vi "Komponente aus Gasflasche ermitteln.vi"(0 "Referenz Gasflasche":refnum<vi>, 1 "Konzentration IST":dbl, 2 "Wertänderung Gasflasche":bool, 5 "Referenz Komponente":refnum<vi>, 9 "Referenz Konfig Gasflasche":refnum<vi>, 11 "error in (no error)":errorcluster caption="Fehler (Eingang, kein Fehler)") -> (4 "Komponente":string, 6 "Bottle Index":T1 caption="Wert" items=["----"=10000, "IAG NH3 3000"=0, "IAG NH3 200"=1, "IAG NH3 2000"=2, "IAG MG"=3, "IAG O2"=4], 10 "Ausgangs-Cluster":T2, 15 "error out":errorcluster caption="Fehler (Ausgang)")   [LabVIEW 2020, in "System Einstellungen V2.lvlib"]
uses:
  System Einstellungen V2.lvlib
  Gasflasche Auswahl.ctl
  Aktion FGV Gasbottledefinition.ctl
  FT-IR/FGV FT-IR Gasliste Aktionen.ctl
  FT-IR/FT-IR.lvlib
  Gaszuordnung AO/Gaszuordnung AO.lvlib
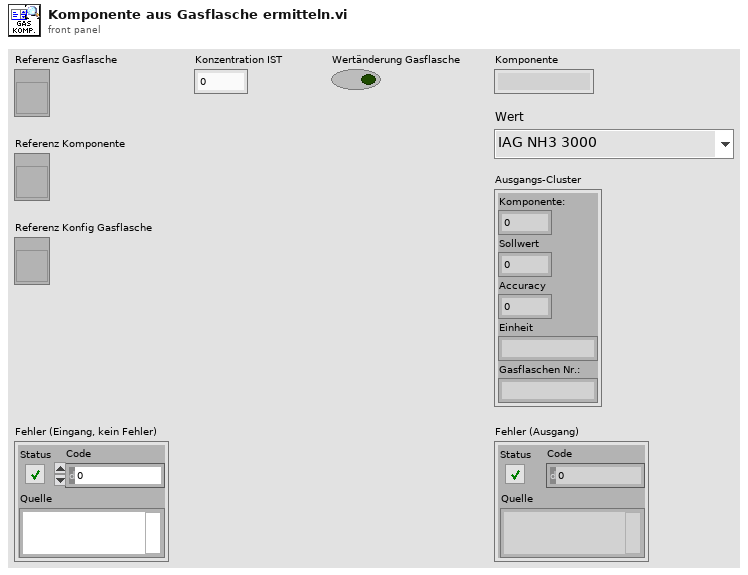
[diagram p1: front panel]
types:
  T1 = typedef "System Einstellungen V2.lvlib/Gasflasche Auswahl.ctl" = u16
  T2 = cluster{"Komponente:":u16, "Sollwert":dbl, "Accuracy":dbl, "Einheit":string, "Gasflaschen Nr.:":string}
  T3 = typedef "FT-IR.lvlib/FGV FT-IR Gasliste Aktionen.ctl" = enum16{"lesen", "Gasliste FT-IR", "Gasliste ausgelesen", "laden", "speichern", "löschen"}
  T4 = typedef "System Einstellungen V2.lvlib/Aktion FGV Gasbottledefinition.ctl" = enum16{"lesen", "schreiben", "löschen", "laden", "speichern", "exportieren", "importieren"}
  T5 = typedef "System Einstellungen V2.lvlib/Gasflasche gesamt.ctl" = cluster{"Gasflasche":T6, "Trägergas":T7, "Komponenten":T8[]}
  T6 = typedef "System Einstellungen V2.lvlib/Gasflasche.ctl" = cluster{"Gasname für die Auswahl":string, "Chargennummer":string, "Ablaufdatum":timestamp}
  T7 = typedef "System Einstellungen V2.lvlib/Traegergas.ctl" = string
  T8 = typedef "System Einstellungen V2.lvlib/Gasflaschenkomponente.ctl" = cluster{"Gasauswahl":string, "Konzentration IST":dbl, "Einheit":string, "Genauigkeit":dbl}
  T9 = typedef "String - Ausgabefeld.ctl" = string
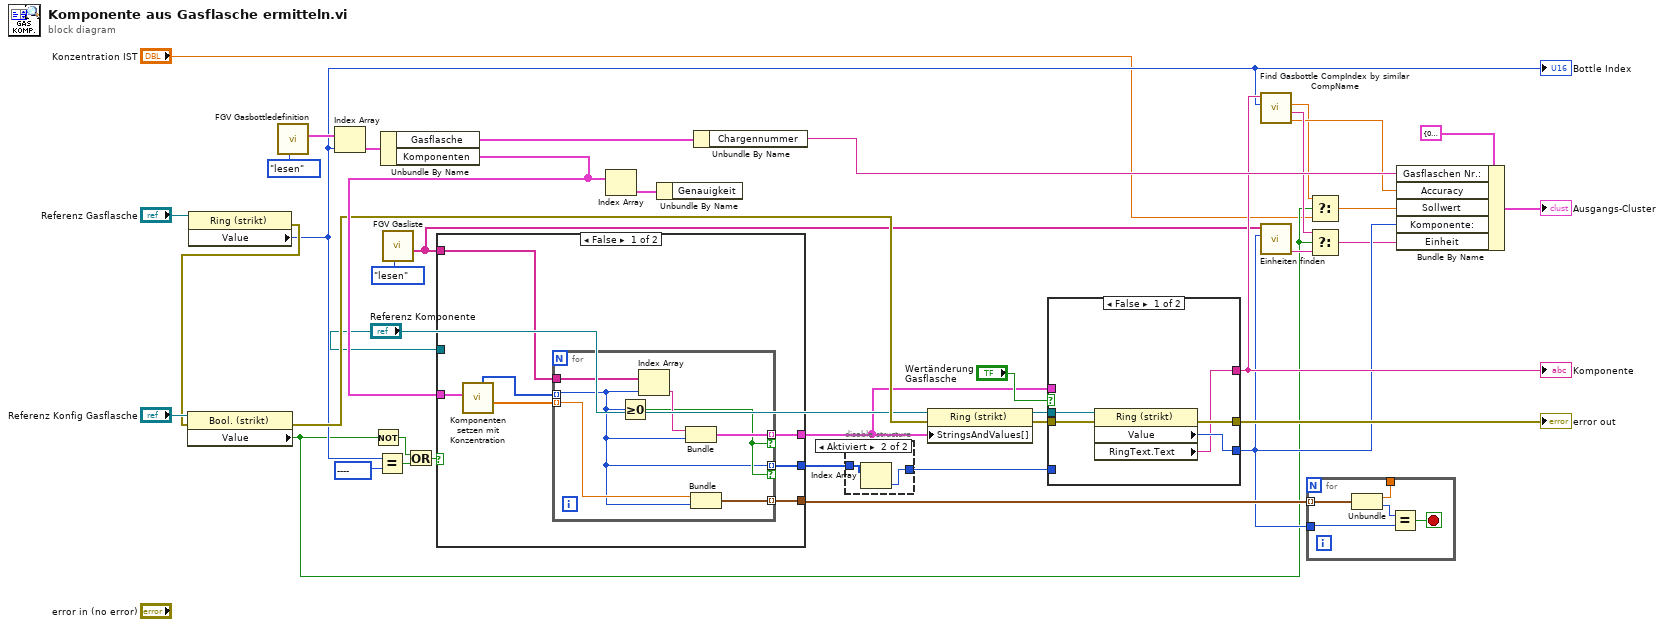
[diagram p0: block diagram]
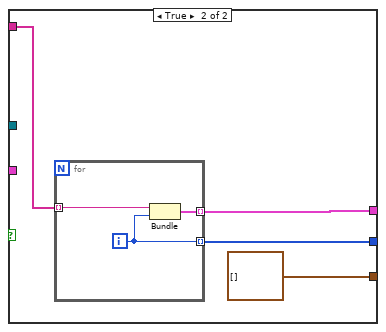
[diagram p2: hidden frame]
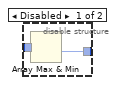
[diagram p3: hidden frame]
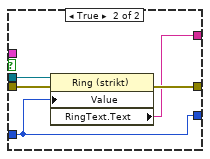
[diagram p4: hidden frame]
diagram:
  w33 = T1 10000 items=["----"=10000, "IAG NH3 3000/2022-11-09/NH3/3000,0000"=0, "IAG NH3 200/2022-11-09/NH3/200,0000"=1, "IAG NH3 2000/2020-12-12/NH3/2000,0000"=2, "IAG MG/2023-08-08/NH3/2000,0000"=3, "IAG O2/2022-11-16/O2/10,0000"=4] ("y")
  n1 = property on="Eigenschaftsknoten" class="Ring (strikt)"(reference="Referenz Gasflasche") -> (error out=w17:errorcluster, "Value"=w13:T1)  [unwired: 1 in, 1 out]
  "Bottle Index" <- w13
  n2 = property on="Eigenschaftsknoten" class="Bool. (strikt)"(reference="Referenz Konfig Gasflasche", error in=w17) -> (error out=w22:errorcluster, "Value"=w4:bool)  [unwired: 1 out]
  n3 = call "FGV Gasbottledefinition.vi"("Aktion"=Aktion_FGV_Gasbottledefinition."lesen") -> ("Gasflaschen Liste gesamt"=w39:T5[])  [unwired: 8 in, 2 out]
  n4 = Index Array(array=w39, index=w13) -> (element=w38:T5)
  n5 = Not(x=w4) -> (.not. x?=w19:bool)
  n6 = Equal?(x=w13, y=w33) -> (x = y?=w21:bool)
  n7 = Unbundle By Name(w38) -> ("Gasflasche"=w36:T6, "Komponenten"=w35:T8[])
  n8 = call "FGV Gasliste.vi"("Aktionen"=FGV_FT-IR_Gasliste_Aktionen."lesen") -> ("Aktuelle Gasliste gesamt"=w10:T9[])  [unwired: 8 in, 2 out]
  n9 = Or(x=w19, y=w21) -> (x .or. y?=w20:bool)
  n10 = case shown="False" w20 {
    tunnel: w35 -> [w42 _]
    tunnel: w10 -> [w46 w57]
    tunnel: [w45 w56] -> w15
    tunnel: [w44 w55] -> w32
    tunnel: [w43 cluster{"Konzentration IST":dbl, i32}[] []] -> w27
    tunnel: "Referenz Komponente" -> [_ _]
    frame False {
      n11 = call "Komponenten setzen mit Konzentration.vi"("Komponenten"=w42) -> ("Konzentrationen"=w41:dbl[], "Indizes"=w40:i32[])  [unwired: 6 in, 3 out]
      n12 = for {
        tunnel: w40 -> [w48] mode=indexing
        tunnel: w46 -> [w53]
        tunnel: [w51] -> w45 mode=indexing if=w50
        tunnel: [w48] -> w44 mode=indexing if=w50
        tunnel: w41 -> [w49] mode=indexing
        tunnel: [w47] -> w43 mode=indexing
        n13 = Greater Or Equal To 0?(x=w48) -> (x >= 0?=w50:bool)
        n14 = Index Array(array=w53, index=w48) -> (element=w52:T9)
        n15 = Bundle("String - Ausgabefeld"=w52, w48) -> (w51:cluster{"String - Ausgabefeld":T9, i32})  [unwired: 1 in]
        n16 = Bundle("Konzentration IST"=w49, w48) -> (w47:cluster{"Konzentration IST":dbl, i32})  [unwired: 1 in]
      }
    }
    frame True {
      n17 = for {
        tunnel: w57 -> [w60] mode=indexing
        tunnel: [w59] -> w56 mode=indexing
        tunnel: [w58] -> w55 mode=indexing
        i -> [w58]
        n18 = Bundle("String - Ausgabefeld"=w60, w58) -> (w59:cluster{"String - Ausgabefeld":T9, i32})  [unwired: 1 in]
      }
    }
  }
  n19 = Index Array(array=w35) -> (element=w37:T8)  [unwired: 1 in]
  n20 = Unbundle By Name(w37) -> ()  [unwired: 1 out]
  n21 = Unbundle By Name(w36) -> ("Chargennummer"=w26:string)
  n22 = disable-structure shown="Aktiviert" {
    disable-tunnel: w32 -> [w62 w64]
    disable-tunnel: [w61 w63] -> w16
    frame Disabled {
      n23 = Array Max & Min(array=w62) -> (min value=w61:i32)  [unwired: 3 out]
    }
    frame Enabled {
      n24 = Index Array(array=w64) -> (element=w63:i32)  [unwired: 1 in]
    }
  }
  n25 = property on="Eigenschaftsknoten" class="Ring (strikt)"(reference="Referenz Komponente", error in=w22, "StringsAndValues[]"=w15) -> (reference out=w29:refnum<vi>, error out=w28:errorcluster)
  n26 = case shown="False" "Wertänderung Gasflasche" {
    tunnel: w29 -> [w69 w74]
    tunnel: w28 -> [w68 w73]
    tunnel: [w67 w72] -> w24
    tunnel: [w66 w71] -> w11
    tunnel: w16 -> [_ w71]
    tunnel: [w65 w70] -> w14
    tunnel: w15 -> [_ _]
    frame False {
      n27 = property on="Eigenschaftsknoten" class="Ring (strikt)"(reference=w69, error in=w68) -> (error out=w67:errorcluster, "Value"=w66:u16, "RingText.Text"=w65:string)  [unwired: 1 out]
    }
    frame True {
      n28 = property on="Eigenschaftsknoten" class="Ring (strikt)"(reference=w74, error in=w73, "Value"=w71) -> (error out=w72:errorcluster, "RingText.Text"=w70:string)  [unwired: 1 out]
    }
  }
  "error out" <- w24
  "Komponente" <- w14
  n29 = call "Find Gasbottle CompIndex by similar CompName.vi"("Botle Index"=w13, "Comp Name"=w14) -> ("Genauigkeit"=w6:dbl, "Einheit"=w12:string, "Konzentration IST"=w3:dbl)  [unwired: 3 in, 4 out]
  n30 = call "Einheiten finden.vi"("Komponente"=w11, "Aktuelle Gasliste gesamt"=w10) -> ("Einheit in String"=w7:string)  [unwired: 8 in, 1 out]
  n31 = for {
    tunnel: w27 -> [w79] mode=indexing
    tunnel: [w78] -> _
    tunnel: w11 -> [w76]
    stop <- w75 stop-if-true
    n32 = Unbundle(w79) -> ("Konzentration IST"=w78:dbl, w77:i32)
    n33 = Equal?(x=w77, y=w76) -> (x = y?=w75:bool)
  }
  n34 = Select(t=w3, s=w4, f="Konzentration IST") -> (s? t:f=w2:dbl)
  n35 = Select(t=w12, s=w4, f=w7) -> (s? t:f=w5:string)
  n36 = Bundle By Name(cluster=T2 {"Komponente:"=0, "Sollwert"=0.0, "Accuracy"=0.0, "Einheit"="", "Gasflaschen Nr.:"=""} ("Ausgangs-Cluster"), "Gasflaschen Nr.:"=w26, "Accuracy"=w6, "Sollwert"=w2, "Komponente:"=w11, "Einheit"=w5) -> (→"Ausgangs-Cluster":T2)
